vi "depth_sweep_smooth.vi"(0 "Frequency":dbl, 1 "Channel (1:Channel 1)":i32, 2 "AD2":i32, 3 "DC Offset (0.00 V)":dbl min=-10.0 max=10.0, 4 "SG Device":T1(ring) caption="Signal Generator Device", 5 "Modulation frequency":dbl, 6 "Current Sweep Value":refnum<vi>, 7 "Delay":dbl, 8 "Start t":refnum<vi>, 9 "Modulation Depth (0.0 %) 2":dbl[](array[numeric]), 11 "error in (no error)":errorcluster, 12 "Siglent Name":refnum<visa-resource-name>="USB0::0xF4EC::0x1102::SDG2XCAD4R3627::INSTR", 13 "Amplitude":dbl, 14 "Stop 2":bool) -> (15 "error out":errorcluster)   [LabVIEW 2024, in "Sweep.lvlib"]
uses:
  Sweep.lvlib
  AD2/Node Parameters.ctl
  <instrlib>/Siglent SDG 1000 5000 800 Series/Public/Configure/Configure Modulation (AM).vi
  <instrlib>/Siglent SDG 1000 5000 800 Series/Siglent SDG 1000 5000 800 Series.lvlib
  AD2/AD2 DLL.lvlib
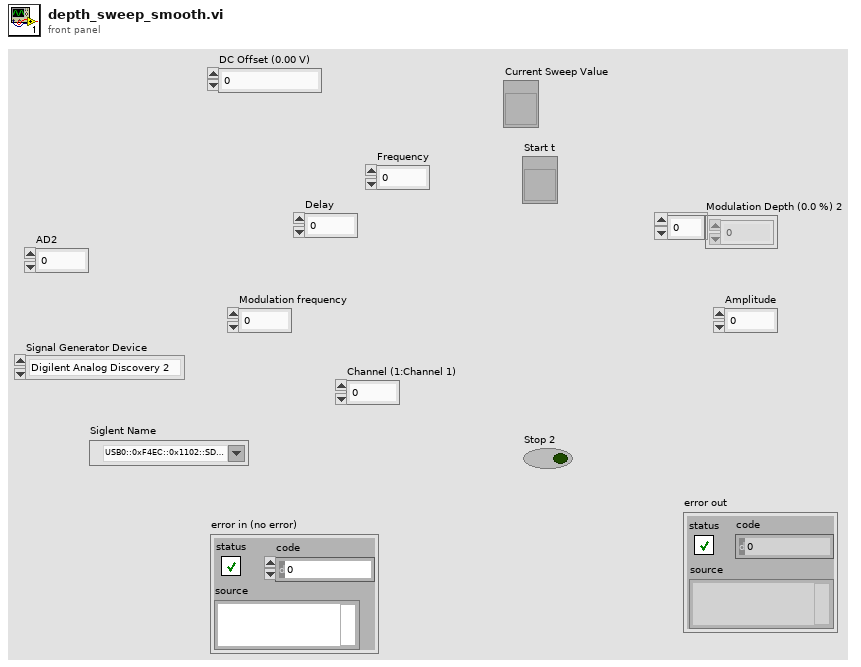
[diagram p1: front panel]
types:
  T1 = enum16{"Digilent Analog Discovery 2", "Siglent DG"}
  T2 = typedef "AD2 DLL.lvlib/Node Parameters.ctl" = cluster{"Function":u8, "Frequency":dbl, "Amplitude":dbl, "DC Offset":dbl, "Duty Cycle":dbl, "Phase":dbl}
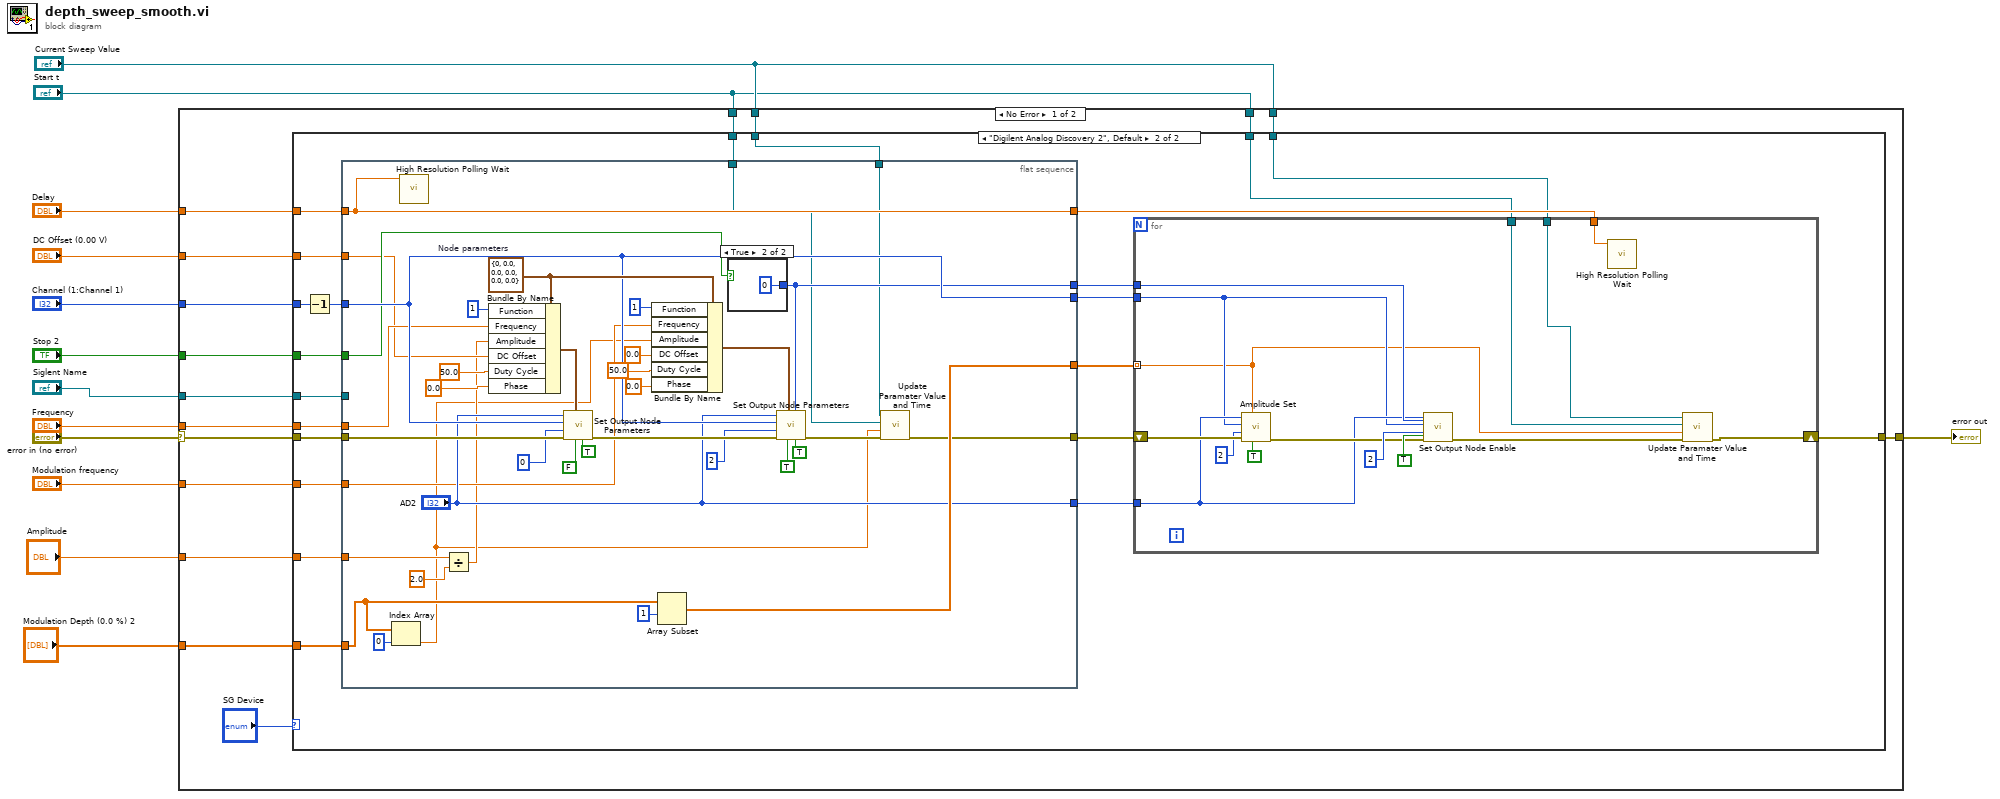
[diagram p0: block diagram]
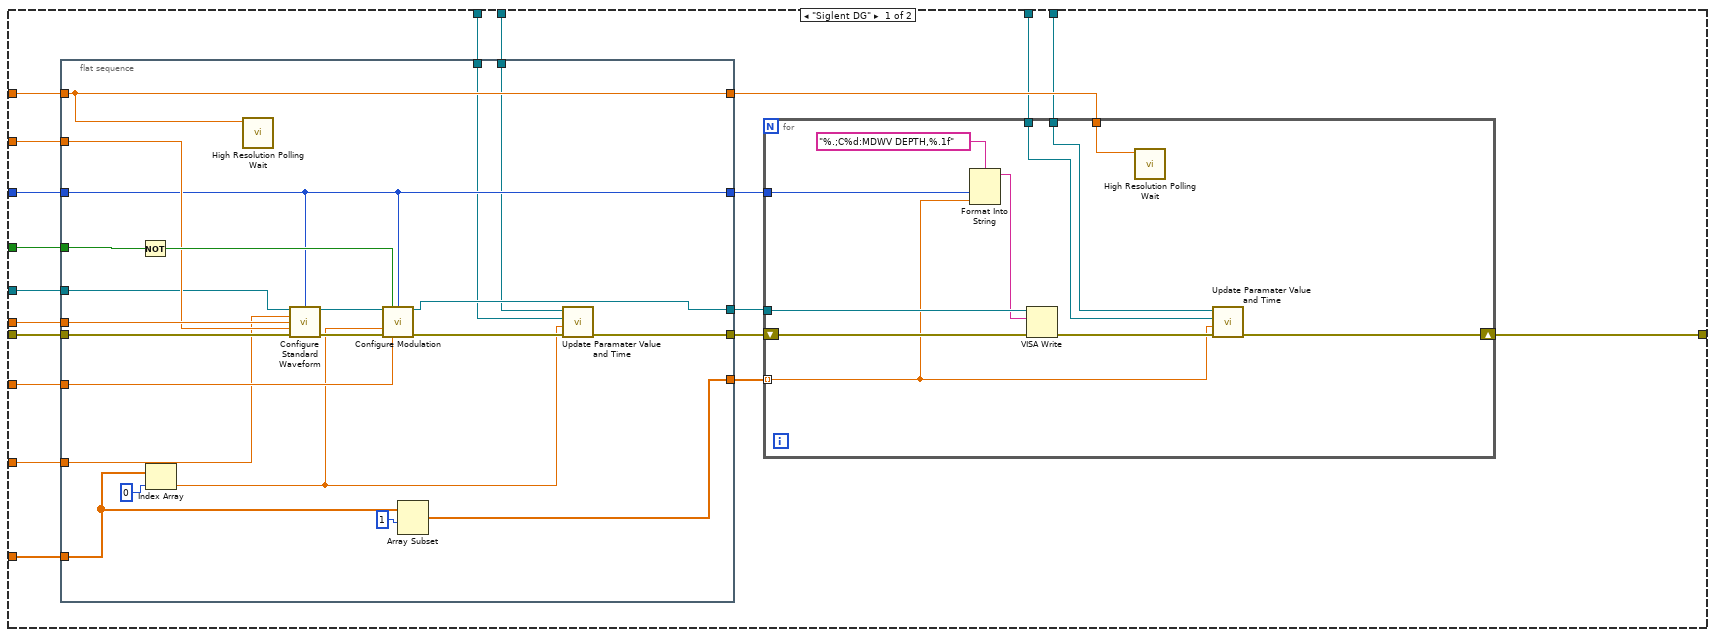
[diagram p2: hidden frame]
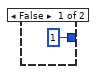
[diagram p3: hidden frame]
diagram:
  n1 = case shown="No Error" "error in (no error)" {
    selector: "error in (no error)" -> [w21 w160]
    tunnel: "Modulation frequency" -> [w29 _]
    tunnel: "Frequency" -> [w28 _]
    tunnel: "Stop 2" -> [w27 _]
    tunnel: [w26 w160] -> w10
    tunnel: "Channel (1:Channel 1)" -> [w25 _]
    tunnel: "Delay" -> [w24 _]
    tunnel: "DC Offset (0.00 V)" -> [w23 _]
    tunnel: "Siglent Name" -> [w22 _]
    tunnel: "Amplitude" -> [w19 _]
    tunnel: "Modulation Depth (0.0 %) 2" -> [w18 _]
    tunnel: "Current Sweep Value" -> [w17 _]
    tunnel: "Current Sweep Value" -> [w16 _]
    tunnel: "Start t" -> [w15 _]
    tunnel: "Start t" -> [w14 _]
    frame No Error {
      n2 = case shown="\"Digilent Analog Discovery 2\", Default" "SG Device" {
        tunnel: w29 -> [w48 w104]
        tunnel: w28 -> [w47 w103]
        tunnel: w27 -> [w46 w102]
        tunnel: [w44 w100] -> w26
        tunnel: w25 -> [w42 w98]
        tunnel: w24 -> [w41 w97]
        tunnel: w23 -> [w40 w96]
        tunnel: w22 -> [w39 w95]
        tunnel: w21 -> [w38 w94]
        tunnel: w19 -> [w35 w88]
        tunnel: w18 -> [w34 w87]
        tunnel: w17 -> [w33 w86]
        tunnel: w16 -> [w32 w85]
        tunnel: w15 -> [w31 w84]
        tunnel: w14 -> [w30 w83]
        frame "Siglent DG" {
          n3 = flat-sequence {
            tunnel: [w70] -> w49
            tunnel: w48 -> [w67]
            tunnel: w47 -> [w66]
            tunnel: w46 -> [w65]
            tunnel: [w53] -> w45
            tunnel: [w62] -> w43
            tunnel: w42 -> [w57]
            tunnel: w41 -> [w58]
            tunnel: w40 -> [w61]
            tunnel: w39 -> [w60]
            tunnel: w38 -> [w59]
            tunnel: [w58] -> w37
            tunnel: [w57] -> w36
            tunnel: w35 -> [w56]
            tunnel: w34 -> [w55]
            tunnel: w32 -> [w51]
            tunnel: w31 -> [w50]
            frame #0 {
              n4 = Not(x=w65) -> (.not. x?=w71:bool)
              n5 = Index Array(array=w55, index=0) -> (element=w52:dbl)
              n6 = call <vilib>:"High Resolution Polling Wait.vi"("seconds to wait"=w58) -> ()  [unwired: 10 in, 1 out]
              n7 = call <instrlib>:"Configure Standard Waveform.vi"("VISA resource name"=w60, "Channel (1:Channel 1)"=w57, "Amplitude (1.0 Vpp)"=w56, "Frequency (1000 Hz)"=w66, "DC Offset (0.00 V)"=w61, "error in (no error)"=w59) -> ("VISA resource name out"=w68:refnum<visa-resource-name>, "error out"=w69:errorcluster)  [unwired: 8 in]
              n8 = call-poly <instrlib>:"Configure Modulation.vi"("VISA resource name"=w68, "Enable Amplitude Modulation (T:Enable)"=w71, "Channel (1:Channel 1)"=w57, "Modulation Depth (0.0 %)"=w52, "error in (no error)"=w69, "Modulation Frequency (100 Hz)"=w67) -> ("VISA resource name out"=w70:refnum<visa-resource-name>, "error out"=w54:errorcluster)  [unwired: 8 in]
              n9 = Array Subset "Array Subset"(array=w55, index=1) -> (w62:dbl[])  [unwired: 1 in]
              n10 = call "Update Paramater Value and Time.vi"("error in (no error)"=w54, "Value"=w52, "Start t"=w50, "Current Sweep Value"=w51) -> ("error out"=w53:errorcluster)  [unwired: 7 in]
            }
          }
          n11 = for {
            shift-right: [w75] -> w44
            shift-left: w45 -> [w78]
            tunnel: w49 -> [w80]
            tunnel: w37 -> [w77]
            tunnel: w43 -> [w74] mode=indexing
            tunnel: w36 -> [w82]
            tunnel: w33 -> [w73]
            tunnel: w30 -> [w72]
            n12 = Format Into String(format string="%.;C%d:MDWV DEPTH,%.1f", w82, w74) -> (resulting string=w79:string)  [unwired: 2 in, 1 out]
            n13 = VISA Write(VISA resource name=w80, write buffer=w79, error in (no error)=w78) -> (error out=w76:errorcluster)  [unwired: 2 out]
            n14 = call <vilib>:"High Resolution Polling Wait.vi"("seconds to wait"=w77) -> ()  [unwired: 10 in, 1 out]
            n15 = call "Update Paramater Value and Time.vi"("error in (no error)"=w76, "Value"=w74, "Start t"=w72, "Current Sweep Value"=w73) -> ("error out"=w75:errorcluster)  [unwired: 7 in]
          }
        }
        frame "Digilent Analog Discovery 2", Default {
          n16 = Decrement(x=w98) -> (x-1=w92:i32)
          n17 = flat-sequence {
            tunnel: w104 -> [w120]
            tunnel: w103 -> [w116]
            tunnel: w102 -> [w122]
            tunnel: [w108] -> w101
            tunnel: [w140] -> w99
            tunnel: w92 -> [w125]
            tunnel: w97 -> [w139]
            tunnel: w96 -> [w115]
            tunnel: w95 -> [_]
            tunnel: w94 -> [w138]
            tunnel: [w139] -> w89
            tunnel: [w125] -> w93
            tunnel: ["AD2"] -> w91
            tunnel: [w114] -> w90
            tunnel: w88 -> [w111]
            tunnel: w87 -> [w110]
            tunnel: w85 -> [w106]
            tunnel: w84 -> [w105]
            frame #0 {
              w129 = T2 {"Function"=0, "Frequency"=0.0, "Amplitude"=0.0, "DC Offset"=0.0, "Duty Cycle"=0.0, "Phase"=0.0}  # Node parameters
              n18 = Index Array(array=w110, index=0) -> (element=w107:dbl)
              n19 = call <vilib>:"High Resolution Polling Wait.vi"("seconds to wait"=w139) -> ()  [unwired: 10 in, 1 out]
              n20 = Divide(x=w111, y=2.0) -> (x/y=w113:dbl)
              n21 = Bundle By Name(cluster=w129, "Function"=u8 1, "Frequency"=w116, "Amplitude"=w113, "DC Offset"=w115, "Duty Cycle"=50.0, "Phase"=0.0) -> (w136:T2)
              n22 = call "Set Output Node Parameters.vi"("Apply parameters"=TRUE, "Use Enable"=FALSE, "Node parameters"=w136, "error in (no error)"=w138, "node"=0, "idxChannel"=w125, "hdwf"="AD2") -> ("error out"=w137:errorcluster)  [unwired: 3 in, 1 out]
              n23 = Bundle By Name(cluster=w129, "Function"=u8 1, "Frequency"=w120, "Amplitude"=w107, "DC Offset"=0.0, "Duty Cycle"=50.0, "Phase"=0.0) -> (w128:T2)
              n24 = Array Subset "Array Subset"(array=w110, index=1) -> (w140:dbl[])  [unwired: 1 in]
              n25 = case shown="True" w122 {
                tunnel: [1 ("Enable") 0 ("Enable")] -> w114
                frame False {
                }
                frame True {
                }
              }
              n26 = call "Set Output Node Parameters.vi"("Apply parameters"=TRUE, "Enable"=w114, "Use Enable"=TRUE, "Node parameters"=w128, "error in (no error)"=w137, "node"=2, "idxChannel"=w125, "hdwf"="AD2") -> ("error out"=w109:errorcluster)  [unwired: 2 in, 1 out]
              n27 = call "Update Paramater Value and Time.vi"("error in (no error)"=w109, "Value"=w107, "Start t"=w105, "Current Sweep Value"=w106) -> ("error out"=w108:errorcluster)  [unwired: 7 in]
            }
          }
          n28 = for {
            shift-right: [w148] -> w100
            shift-left: w101 -> [w155]
            tunnel: w99 -> [w145] mode=indexing
            tunnel: w93 -> [w152]
            tunnel: w91 -> [w153]
            tunnel: w90 -> [w158]
            tunnel: w89 -> [w157]
            tunnel: w86 -> [w147]
            tunnel: w83 -> [w146]
            n29 = call "Amplitude Set.vi"("Update"=TRUE, "Amplitude"=w145, "error in (no error)"=w155, "node"=2, "idxChannel"=w152, "hdwf"=w153) -> ("error out"=w154:errorcluster)  [unwired: 3 in, 2 out]
            n30 = call "Set Output Node Enable.vi"("Update"=TRUE, "Enable"=w158, "error in (no error)"=w154, "node"=2, "idxChannel"=w152, "hdwf"=w153) -> ("error out"=w149:errorcluster)  [unwired: 4 in, 1 out]
            n31 = call <vilib>:"High Resolution Polling Wait.vi"("seconds to wait"=w157) -> ()  [unwired: 10 in, 1 out]
            n32 = call "Update Paramater Value and Time.vi"("error in (no error)"=w149, "Value"=w145, "Start t"=w146, "Current Sweep Value"=w147) -> ("error out"=w148:errorcluster)  [unwired: 7 in]
          }
        }
      }
    }
    frame Error {
    }
  }
  "error out" <- w10
